vi "pathhandler.vi"() -> ()   [LabVIEW 2020]
uses:
  <vilib>/Rock Robotics/WPI/ThirdParty/JAS_Junk/TrajLib/Trajectory_Library.lvlib
  Robot Global Data.vi
  <vilib>/Rock Robotics/WPI/ThirdParty/JAS_Junk/TrajLib/TypeDef/TRANSLATION2D.ctl
  <vilib>/Rock Robotics/WPI/ThirdParty/JAS_Junk/TrajLib/TypeDef/ROTATION2D.ctl
  <vilib>/Rock Robotics/WPI/ThirdParty/JAS_Junk/TrajLib/TypeDef/POSE2D.ctl
  <vilib>/Rock Robotics/WPI/ThirdParty/JAS_Junk/TrajLib/TypeDef/TRAJ_STATE.ctl
  <vilib>/Rock Robotics/WPI/ThirdParty/JAS_Junk/TrajLib/TypeDef/CHASSIS_SPEEDS.ctl
  <vilib>/Rock Robotics/WPI/ThirdParty/JAS_Junk/TrajLib/TypeDef/TRAJECTORY.ctl
panel:
  in  "traj input":T1 {"States"."POSE"."ROTATION"."SIN" format="%13.4f"; "States"."POSE"."ROTATION"."COS" format="%13.4f"; "States"."POSE"."ROTATION"."VALUE" format="%13.4f"; "States"."POSE"."TRANSLATION"."Y" format="%14.3f"; "States"."POSE"."TRANSLATION"."X" format="%14.3f"; "TotalTImeSecs" format="%20.3f"}
  in  "AttainableMaxSpeed":dbl
  out "Error and Corr":T6 {"Error Pose"."ROTATION"."SIN" format="%13.4f"; "Error Pose"."ROTATION"."COS" format="%13.4f"; "Error Pose"."ROTATION"."VALUE" format="%13.4f"; "Error Pose"."TRANSLATION"."Y" format="%14.3f"; "Error Pose"."TRANSLATION"."X" format="%14.3f"}
  in  "Time Offset":dbl=-1.0 format="%16.4f"
  in  "EnableClosedLoop":bool=TRUE
  out "Chassis Velocity Target":T7 {"vOmega" format="%10.3f"; "vY" format="%10.3f"; "vX" format="%10.3f"}
  out "OutputTRAJ_STATE":T2={"TimeSeconds"=0.0, "Velocity"=0.0, "Acceleration"=0.0, "POSE"={"TRANSLATION"={"X"=0.0, "Y"=0.0}, "ROTATION"={"VALUE"=0.0, "COS"=1.0, "SIN"=0.0}}, "Curvature"=0.0} {"POSE"."ROTATION"."SIN" format="%13.4f"; "POSE"."ROTATION"."COS" format="%13.4f"; "POSE"."ROTATION"."VALUE" format="%13.4f"; "POSE"."TRANSLATION"."Y" format="%14.3f"; "POSE"."TRANSLATION"."X" format="%14.3f"}
  in  "Orientation Dmd In":dbl
  out "Orientation Target":dbl
  in  "Reverse":bool
  in  "Follow Orientation":bool
  in  "Gyro Heading":dbl
  out "AtReference":bool
  in  "Init":bool
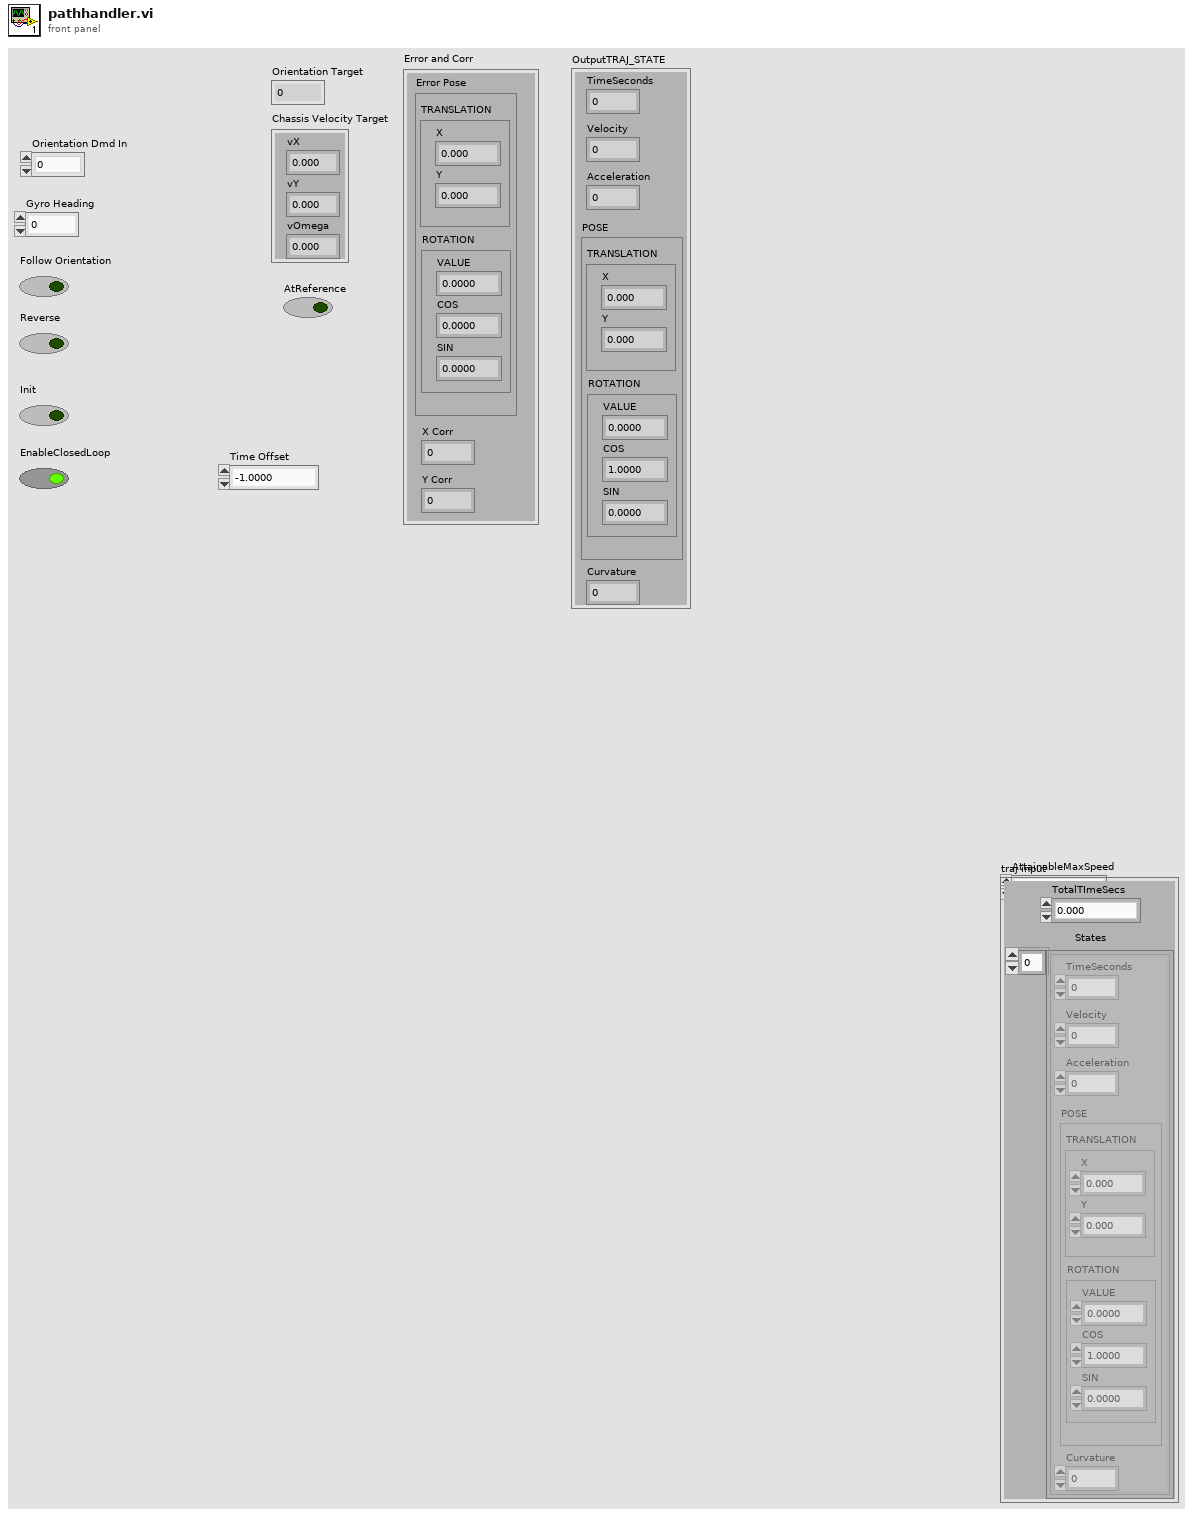
[diagram p1: front panel]
types:
  T1 = typedef "Trajectory_Library.lvlib/TRAJECTORY.ctl" = cluster{"TotalTImeSecs":dbl, "States":T2[]}
  T2 = typedef "Trajectory_Library.lvlib/TRAJ_STATE.ctl" = cluster{"TimeSeconds":dbl, "Velocity":dbl, "Acceleration":dbl, "POSE":T3, "Curvature":dbl}
  T3 = typedef "Trajectory_Library.lvlib/POSE2D.ctl" = cluster{"TRANSLATION":T4, "ROTATION":T5}
  T4 = typedef "Trajectory_Library.lvlib/TRANSLATION2D.ctl" = cluster{"X":dbl, "Y":dbl}
  T5 = typedef "Trajectory_Library.lvlib/ROTATION2D.ctl" = cluster{"VALUE":dbl, "COS":dbl, "SIN":dbl}
  T6 = cluster{"Error Pose":T3, "X Corr":dbl, "Y Corr":dbl}
  T7 = typedef "Trajectory_Library.lvlib/CHASSIS_SPEEDS.ctl" = cluster{"vX":dbl, "vY":dbl, "vOmega":dbl}
  T8 = typedef "Trajectory_Library.lvlib/SWERVE_DRIVE_KINEMATICS.ctl" = cluster{"NumModules":i32, "InverseKinematics":T9, "ForwardKinematics":T9, "Modules":T4[], "PrevCoR":T4, "SavedModuleStates":T10[]}
  T9 = typedef "NI_Matrix.lvlib/RealMatrix.ctl" = dbl[][]
  T10 = typedef "Trajectory_Library.lvlib/SWERVE_DRIVE_MODULE_STATE.ctl" = cluster{"Speed":dbl, "Angle":T5}
  T11 = typedef "Trajectory_Library.lvlib/SWERVE_DRIVE_MODULE_POSITION.ctl" = cluster{"Distance":dbl, "Angle":T5, "P":bool}
  T12 = typedef "Trajectory_Library.lvlib/SWERVE_DRIVE_ODOMETRY.ctl" = cluster{"POSE":T3, "GyroOffset":T5, "PreviousAngle":T5, "PrevModulePositions":T11[], "NumModules":i32}
  T13 = typedef "Trajectory_Library.lvlib/PID_TUNING.ctl" = cluster{"Kp":dbl, "Ki":dbl, "Kd":dbl, "MaximumIntegral":dbl, "MinimumIntegral":dbl}
  T14 = typedef "Trajectory_Library.lvlib/PID_ERROR_TOLERANCE.ctl" = cluster{"PositionTolerance":dbl, "VelocityTolerance":dbl}
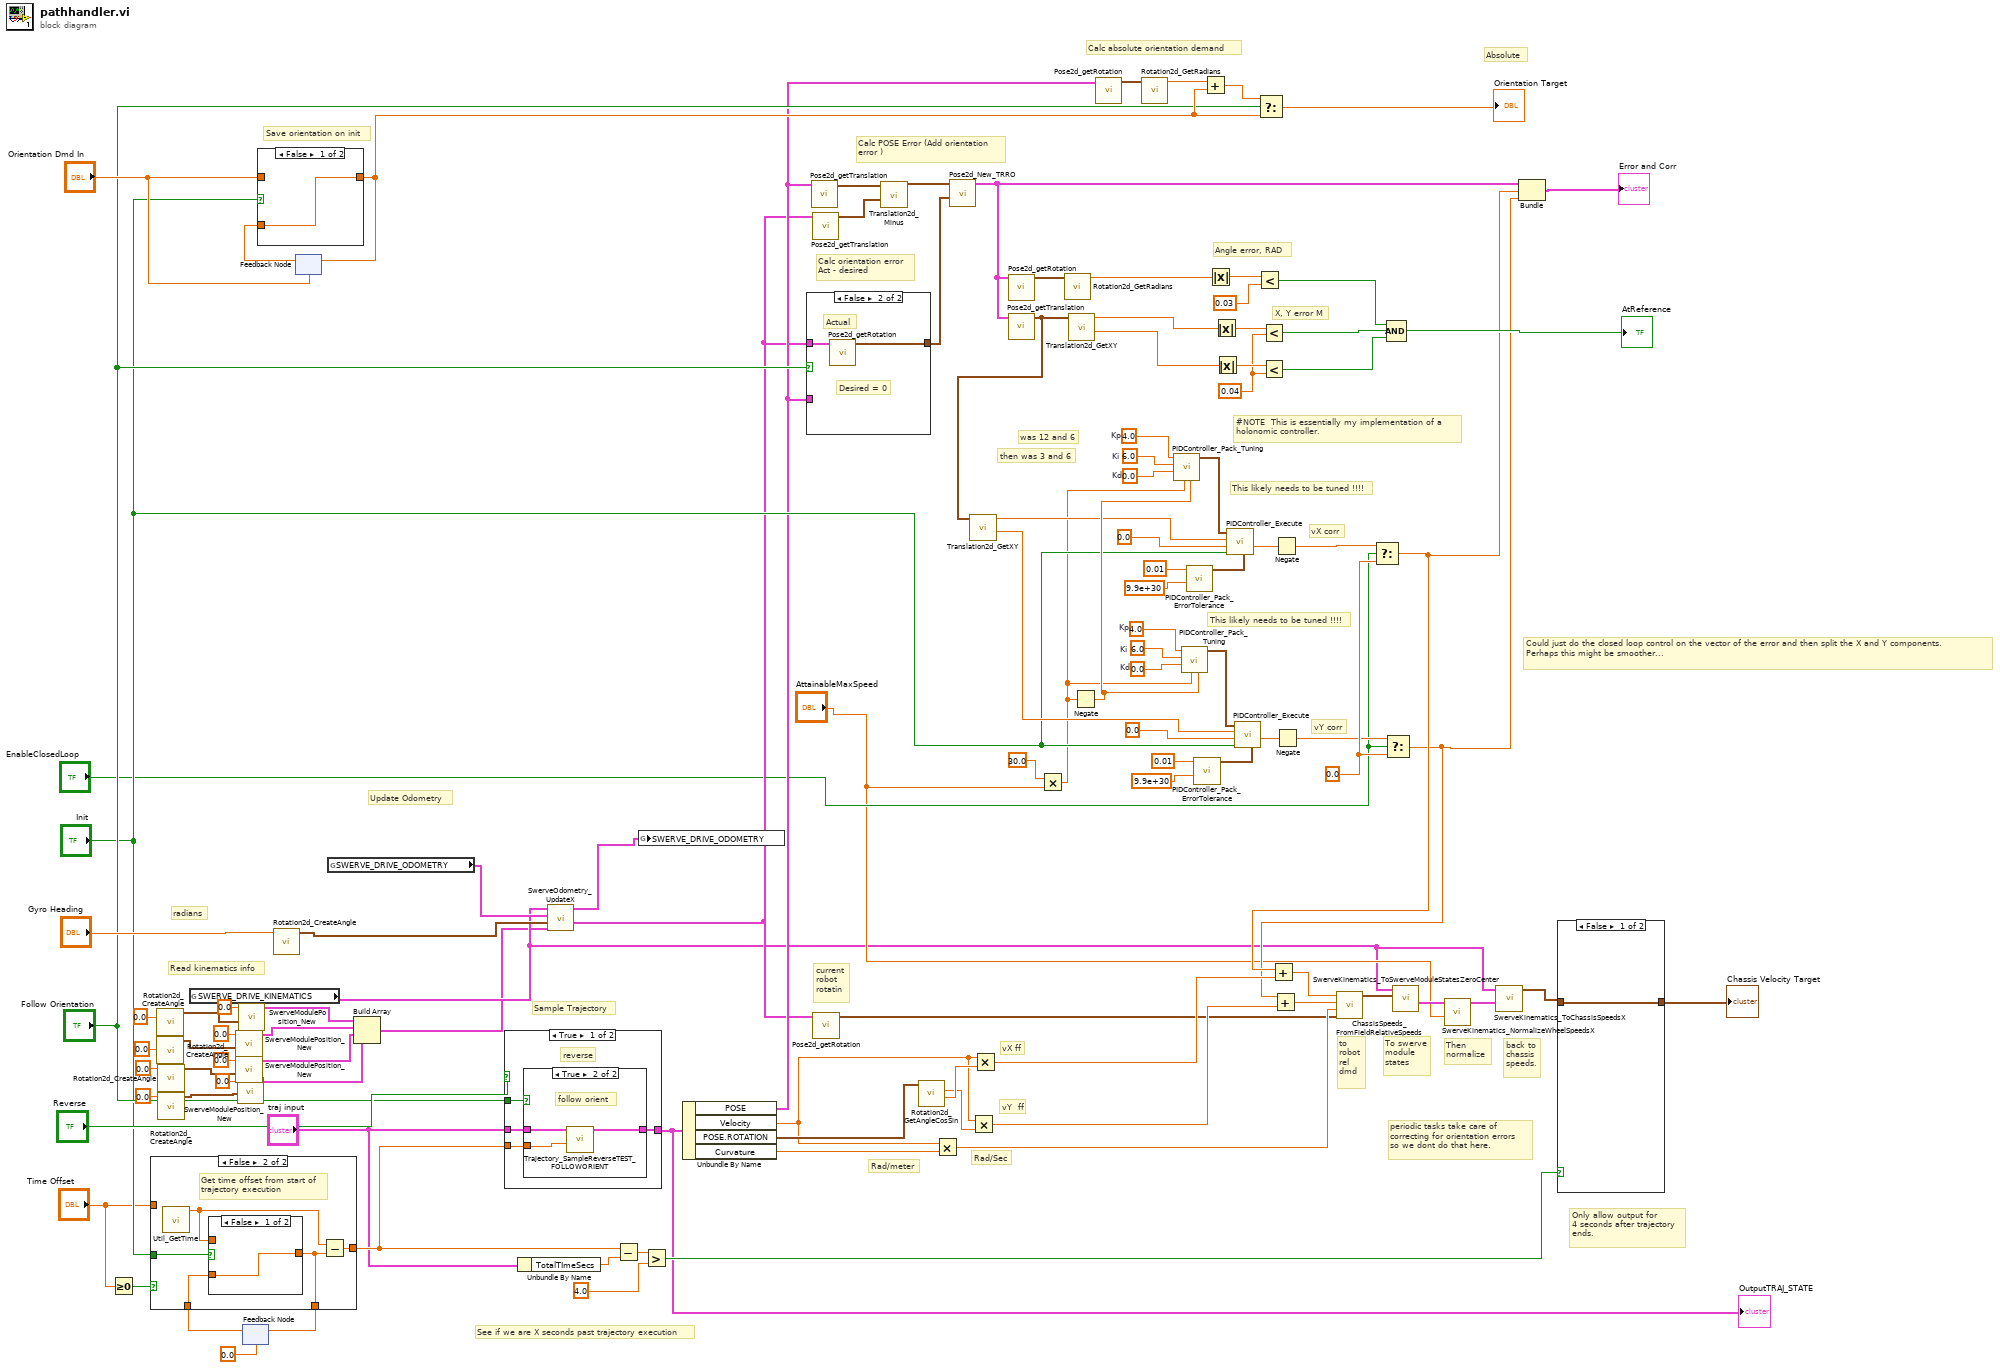
[diagram p0: block diagram]
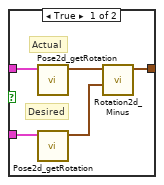
[diagram p4: hidden frame]
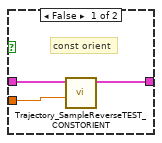
[diagram p5: hidden frame]
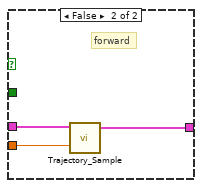
[diagram p6: hidden frame]
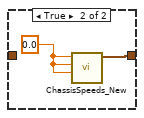
[diagram p8: hidden frame]
diagram:
  w63 = 0.0  # Kd
  w64 = 6.0  # Ki
  w65 = 4.0  # Kp
  w72 = 0.0  # Kd
  w73 = 6.0  # Ki
  w74 = 4.0  # Kp
  w82 = 0.0 ("f")
  w101 = 0.04
  # "#NOTE  This is essentially my implementation of a\nholonomic controller."
  # "Angle error, RAD"
  # "X, Y error M"
  # "then was 3 and 6"
  # "was 12 and 6"
  # "to\nrobot\nrel\ndmd"
  # "This likely needs to be tuned !!!!"
  # "This likely needs to be tuned !!!!"
  # "Could just do the closed loop control on the vector of the error and then split the X and Y components.  \nPerhaps this might be smoother..."
  # "vY corr"
  # "vX corr"
  # "current\nrobot\nrotatin"
  # "vY  ff"
  # "vX ff"
  # "back to\nchassis\nspeeds."
  # "Then\nnormalize"
  # "To swerve\nmodule\nstates"
  # "Rad/Sec"
  # "Rad/meter"
  # "Calc POSE Error (Add orientation\nerror )"
  # "Calc orientation error\nAct - desired"
  # "Calc absolute orientation demand"
  # "Read kinematics info"
  # "Sample Trajectory"
  # "See if we are X seconds past trajectory execution"
  # "Save orientation on init"
  # "Absolute"
  # "Update Odometry"
  # "radians"
  # "periodic tasks take care of\ncorrecting for orientation errors\nso we dont do that here."
  # "Only allow output for\n4 seconds after trajectory\nends."
  n1 = Greater Or Equal To 0?(x="Time Offset") -> (x >= 0?=w30:bool)
  n2 = call <vilib>:"Rotation2d_CreateAngle.vi"("Angle"=0.0) -> ("ROTATION"=w8:T5)  [unwired: 10 in]
  n3 = call <vilib>:"Rotation2d_CreateAngle.vi"("Angle"=0.0) -> ("ROTATION"=w7:T5)  [unwired: 10 in]
  n4 = call <vilib>:"Rotation2d_CreateAngle.vi"("Angle"=0.0) -> ("ROTATION"=w6:T5)  [unwired: 10 in]
  n5 = call <vilib>:"Rotation2d_CreateAngle.vi"("Angle"=0.0) -> ("ROTATION"=w5:T5)  [unwired: 10 in]
  n6 = global read "Robot Global Data.vi" "SWERVE_DRIVE_KINEMATICS"() -> (w18:T8)
  n7 = call <vilib>:"SwerveModulePosition_New.vi"("ROTATION"=w7, "Distance"=0.0) -> ("SWERVE_DRIVE_MODULE_POSITION"=w15:T11)  [unwired: 9 in]
  n8 = call <vilib>:"SwerveModulePosition_New.vi"("ROTATION"=w6, "Distance"=0.0) -> ("SWERVE_DRIVE_MODULE_POSITION"=w14:T11)  [unwired: 9 in]
  n9 = call <vilib>:"SwerveModulePosition_New.vi"("ROTATION"=w5, "Distance"=0.0) -> ("SWERVE_DRIVE_MODULE_POSITION"=w13:T11)  [unwired: 9 in]
  n10 = call <vilib>:"SwerveModulePosition_New.vi"("ROTATION"=w8, "Distance"=0.0) -> ("SWERVE_DRIVE_MODULE_POSITION"=w17:T11)  [unwired: 9 in]
  n11 = feedback #1(0.0 ("TIME")) -> (w32:dbl)
  n12 = case shown="False" w30 {
    tunnel: [w113 w119] -> w111
    tunnel: "Init" -> [_ w117]
    tunnel: w32 -> [w114 w116]
    tunnel: [w114 w115] -> w31
    tunnel: "Time Offset" -> [w113 _]
    frame True {
      # "For testing allow\nuser entered time offset!!"
    }
    frame False {
      # "Get time offset from start of\ntrajectory execution"
      n13 = call <vilib>:"Util_GetTime.vi"() -> ("FPGA_Time_Seconds"=w118:dbl)  [unwired: 9 in, 2 out]
      n14 = case shown="False" w117 {
        tunnel: [w120 w121] -> w115
        tunnel: w116 -> [w120 _]
        tunnel: w118 -> [_ w121]
        frame False {
        }
        frame True {
        }
      }
      n15 = Subtract(x=w118, y=w115) -> (x-y=w119:dbl)
    }
  }
  n16 = feedback-in #1(w31) -> ()
  n17 = call <vilib>:"Rotation2d_CreateAngle.vi"("Angle"="Gyro Heading") -> ("ROTATION"=w24:T5)  [unwired: 10 in]
  n18 = feedback #2("Orientation Dmd In") -> (w93:dbl)
  n19 = case shown="False" "Init" {
    tunnel: "Orientation Dmd In" -> [_ w123]
    tunnel: [w122 w123] -> w90
    tunnel: w93 -> [w122 _]
    frame False {
    }
    frame True {
    }
  }
  n20 = feedback-in #2(w90) -> ()
  n21 = global read "Robot Global Data.vi" "SWERVE_DRIVE_ODOMETRY"() -> (w19:T12)
  n22 = Build Array(w17, w15, w14, w13) -> (w16:T11[])
  n23 = case shown="True" "Reverse" {
    tunnel: "traj input" -> [w127 w136]
    tunnel: w111 -> [w125 w135]
    tunnel: [w126 w134] -> w106
    tunnel: "Follow Orientation" -> [w124 _]
    frame True {
      # "reverse"
      n24 = case shown="True" w124 {
        tunnel: w127 -> [w130 w133]
        tunnel: [w128 w132] -> w126
        tunnel: w125 -> [w129 w131]
        frame False {
          # "const orient"
          n25 = call "Trajectory_SampleReverseTEST_CONSTORIENT.vi"("Time"=w129, "InputTRAJECTORY"=w130) -> ("OutputTRAJ_STATE"=w128:T2)  [unwired: 9 in]
        }
        frame True {
          # "follow orient"
          n26 = call "Trajectory_SampleReverseTEST_FOLLOWORIENT.vi"("Time"=w131, "InputTRAJECTORY"=w133) -> ("OutputTRAJ_STATE"=w132:T2)  [unwired: 9 in]
        }
      }
    }
    frame False {
      # "forward"
      n27 = call <vilib>:"Trajectory_Sample.vi"("Time"=w135, "InputTRAJECTORY"=w136) -> ("OutputTRAJ_STATE"=w134:T2)  [unwired: 9 in]
    }
  }
  "OutputTRAJ_STATE" <- w106
  n28 = Unbundle By Name("traj input") -> ("TotalTImeSecs"=w112:dbl)
  n29 = call <vilib>:"SwerveOdometry_UpdateX.vi"("module Positions"=w16, "gyroAngle"=w24, "in SWERVE_DRIVE_ODOMETRY"=w19, "SWERVE_DRIVE_KINEMATICS"=w18) -> ("robot POSE"=w38:T3, "out SWERVE_DRIVE_ODOMETRY"=w20:T12)  [unwired: 5 in, 1 out]
  n30 = Subtract(x=w111, y=w112) -> (x-y=w110:dbl)
  n31 = global write "Robot Global Data.vi" "SWERVE_DRIVE_ODOMETRY"(w20) -> ()
  n32 = Greater?(x=w110, y=4.0) -> (0:w108:bool)
  n33 = Unbundle By Name(w106) -> ("POSE"=w39:T3, "Velocity"=w48:dbl, "POSE.ROTATION"=w51:T5, "Curvature"=w86:dbl)
  n34 = case shown="False" "Follow Orientation" {
    tunnel: w38 -> [w141 w143]
    tunnel: w39 -> [w140 _]
    tunnel: [w137 w142] -> w83
    frame True {
      # "Desired"
      # "Actual"
      n35 = call <vilib>:"Pose2d_getRotation.vi"("in POSE"=w141) -> ("out ROTATION"=w139:T5)  [unwired: 10 in]
      n36 = call <vilib>:"Pose2d_getRotation.vi"("in POSE"=w140) -> ("out ROTATION"=w138:T5)  [unwired: 10 in]
      n37 = call <vilib>:"Rotation2d_Minus.vi"("other ROTATION"=w138, "in ROTATION"=w139) -> ("out ROTATION"=w137:T5)  [unwired: 9 in]
    }
    frame False {
      # "Desired = 0"
      # "Actual"
      n38 = call <vilib>:"Pose2d_getRotation.vi"("in POSE"=w143) -> ("out ROTATION"=w142:T5)  [unwired: 10 in]
    }
  }
  n39 = call <vilib>:"Pose2d_getTranslation.vi"("in POSE"=w39) -> ("outTRANSLATION"=w37:T4)  [unwired: 10 in]
  n40 = call <vilib>:"Pose2d_getTranslation.vi"("in POSE"=w38) -> ("outTRANSLATION"=w36:T4)  [unwired: 10 in]
  n41 = call <vilib>:"Pose2d_getRotation.vi"("in POSE"=w38) -> ("out ROTATION"=w41:T5)  [unwired: 10 in]
  n42 = call <vilib>:"Translation2d_Minus.vi"("other Translation"=w36, "In Translation"=w37) -> ("Out Translation"=w35:T4)  [unwired: 9 in]
  n43 = call <vilib>:"Rotation2d_GetAngleCosSin.vi"("in ROTATION"=w51) -> ("Cosine"=w50:dbl, "Sine"=w49:dbl)  [unwired: 8 in, 1 out]
  n44 = Multiply(x=w48, y=w86) -> (x*y=w42:dbl)
  n45 = call <vilib>:"Pose2d_New_TRRO.vi"("ROTATION"=w83, "TRANSLATION"=w35) -> ("outPOSE"=w28:T3)  [unwired: 9 in]
  n46 = Multiply(x=w48, y=w49) -> (x*y=w47:dbl)
  n47 = Multiply(x=w48, y=w50) -> (x*y=w46:dbl)
  n48 = call <vilib>:"Pose2d_getRotation.vi"("in POSE"=w28) -> ("out ROTATION"=w78:T5)  [unwired: 10 in]
  n49 = call <vilib>:"Pose2d_getTranslation.vi"("in POSE"=w28) -> ("outTRANSLATION"=w45:T4)  [unwired: 10 in]
  n50 = call <vilib>:"Translation2d_GetXY.vi"("In Translation"=w45) -> ("Y"=w58:dbl, "X"=w59:dbl)  [unwired: 9 in]
  n51 = Multiply(x=30.0, y="AttainableMaxSpeed") -> (x*y=w52:dbl)
  n52 = call <vilib>:"Rotation2d_GetRadians.vi"("in ROTATION"=w78) -> ("AngleRadians"=w80:dbl)  [unwired: 10 in]
  n53 = call <vilib>:"Translation2d_GetXY.vi"("In Translation"=w45) -> ("Y"=w79:dbl, "X"=w81:dbl)  [unwired: 9 in]
  n54 = Negate(x=w52) -> (-x=w60:dbl)
  n55 = call <vilib>:"Pose2d_getRotation.vi"("in POSE"=w39) -> ("out ROTATION"=w91:T5)  [unwired: 10 in]
  n56 = call <vilib>:"Rotation2d_GetRadians.vi"("in ROTATION"=w91) -> ("AngleRadians"=w89:dbl)  [unwired: 10 in]
  n57 = call <vilib>:"PIDController_Pack_Tuning.vi"("MinimumIntegral"=w60, "MaximumIntegral"=w52, "Kd"=w72, "Ki"=w73, "Kp"=w74) -> ("PID Tuning"=w77:T13)  [unwired: 6 in]
  n58 = call <vilib>:"PIDController_Pack_Tuning.vi"("MinimumIntegral"=w60, "MaximumIntegral"=w52, "Kd"=w63, "Ki"=w64, "Kp"=w65) -> ("PID Tuning"=w68:T13)  [unwired: 6 in]
  n59 = call <vilib>:"PIDController_Pack_ErrorTolerance.vi"("VelocityTolerance"=9.9e+30, "PositionTolerance"=0.01) -> ("PID Error Tolerance"=w75:T14)  [unwired: 9 in]
  n60 = call <vilib>:"PIDController_Pack_ErrorTolerance.vi"("VelocityTolerance"=9.9e+30, "PositionTolerance"=0.01) -> ("PID Error Tolerance"=w66:T14)  [unwired: 9 in]
  n61 = Add(x=w89, y=w90) -> (x+y=w88:dbl)
  n62 = Absolute Value(x=w80) -> (abs(x)=w105:dbl)
  n63 = Absolute Value(x=w81) -> (abs(x)=w104:dbl)
  n64 = Absolute Value(x=w79) -> (abs(x)=w103:dbl)
  n65 = call <vilib>:"PIDController_Execute.vi"("PID Error Tolerance"=w75, "Reset"="Init", "SP-SetPoint"=0.0, "PV-Measurement"=w59, "PID Tuning"=w77) -> ("CO-ControlOutput"=w57:dbl)  [unwired: 4 in, 2 out]
  n66 = call <vilib>:"PIDController_Execute.vi"("PID Error Tolerance"=w66, "Reset"="Init", "SP-SetPoint"=0.0, "PV-Measurement"=w58, "PID Tuning"=w68) -> ("CO-ControlOutput"=w56:dbl)  [unwired: 4 in, 2 out]
  n67 = Less?(x=w105, y=0.03) -> (x < y?=w100:bool)
  n68 = Select(t=w88, s="Follow Orientation", f=w90) -> (s? t:f=→"Orientation Target":dbl)
  n69 = Less?(x=w104, y=w101) -> (x < y?=w99:bool)
  n70 = Less?(x=w103, y=w101) -> (x < y?=w98:bool)
  n71 = Negate(x=w57) -> (-x=w55:dbl)
  n72 = Negate(x=w56) -> (-x=w54:dbl)
  n73 = Select(t=w55, s="EnableClosedLoop", f=w82) -> (s? t:f=w27:dbl)
  n74 = Add(x=w27, y=w46) -> (x+y=w44:dbl)
  n75 = Select(t=w54, s="EnableClosedLoop", f=w82) -> (s? t:f=w26:dbl)
  n76 = Add(x=w26, y=w47) -> (x+y=w43:dbl)
  n77 = call <vilib>:"ChassisSpeeds_FromFieldRelativeSpeeds.vi"("RobotAngle"=w41, "Omega"=w42, "vY"=w43, "vX"=w44) -> ("CHASSIS"=w40:T7)  [unwired: 7 in]
  n78 = Compound Arithmetic op=AND(w100, w99, w98) -> (→"AtReference":bool)
  n79 = call <vilib>:"SwerveKinematics_ToSwerveModuleStatesZeroCenter.vi"("ChassisSpeeds"=w40, "in SWERVE_DRIVE_KINEMATICS"=w18) -> ("ModuleStates"=w96:T10[])  [unwired: 8 in, 1 out]
  n80 = call <vilib>:"SwerveKinematics_NormalizeWheelSpeedsX.vi"("AttainableMaxSpeed"="AttainableMaxSpeed", "in WheelStates"=w96) -> ("out WheelStates"=w95:T10[])  [unwired: 9 in]
  n81 = call <vilib>:"SwerveKinematics_ToChassisSpeedsX.vi"("WheelStates"=w95, "in SWERVE_DRIVE_KINEMATICS"=w18) -> ("Chassis Speed"=w23:T7)  [unwired: 9 in]
  n82 = Bundle("outPOSE"=w28, "f"=w27, "f"=w26) -> (→"Error and Corr":cluster{"outPOSE":T3, "f":dbl, "f":dbl})  [unwired: 1 in]
  n83 = case shown="False" w108 {
    tunnel: w23 -> [w144 _]
    tunnel: [w144 w145] -> w84
    frame False {
    }
    frame True {
      w146 = 0.0 ("vX")
      n84 = call <vilib>:"ChassisSpeeds_New.vi"("vAngular"=w146, "vY"=w146, "vX"=w146) -> ("CHASSIS"=w145:T7)  [unwired: 8 in]
    }
  }
  "Chassis Velocity Target" <- w84
